vi "Voltage-Trans Converter.vi"(8 "Input":dbl, 9 "VoltageTransmissionArray":dbl[][](array[numeric]), 11 "Input":enum16{"Transmission", "Voltage"}(ring)) -> (1 "NearestTransmission":dbl, 3 "NearestVoltage":dbl)   [LabVIEW 2020]
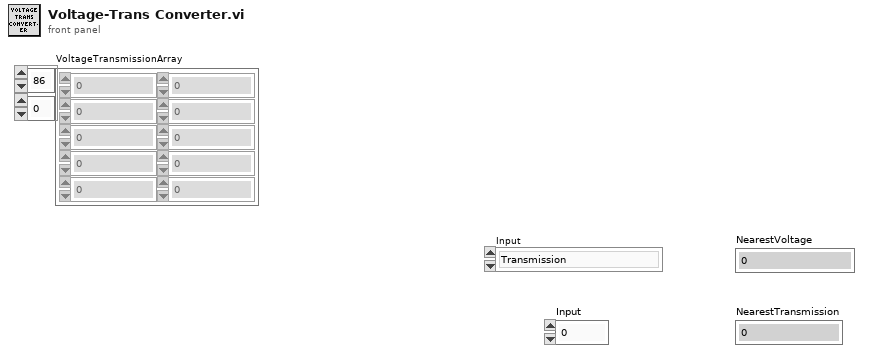
[diagram p1: front panel]
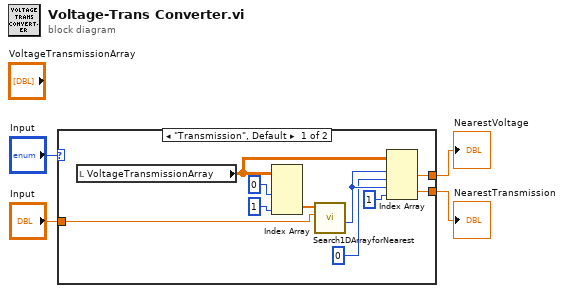
[diagram p0: block diagram]
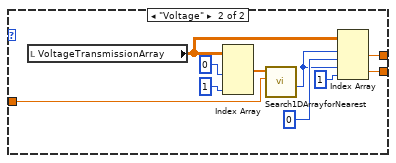
[diagram p2: hidden frame]
diagram:
  n1 = case shown="\"Transmission\", Default" "Input" {
    tunnel: "Input" -> [w8 w21]
    tunnel: [w7 w16] -> w1
    tunnel: [w6 w15] -> w2
    frame "Transmission", Default {
      n2 = local read "VoltageTransmissionArray"() -> (w14:dbl[][])
      n3 = Index Array(array=w14, index (col) #1=0 ("disabled index (col)"), index (col) #2=1 ("index (col)")) -> (element #2=w5:dbl[])  [unwired: 2 in, 1 out]
      n4 = call "Search1DArrayforNearest.vi"("desired element"=w8, "1D Array"=w5) -> ("closest index"=w13:i32)  [unwired: 8 in, 1 out]
      n5 = Index Array(array=w14, index (row) #1=w13, index (col) #1=0 ("disabled index (col)"), index (row) #2=w13, index (col) #2=1 ("index (col)")) -> (element #1=w7:dbl, element #2=w6:dbl)
    }
    frame "Voltage" {
      n6 = local read "VoltageTransmissionArray"() -> (w20:dbl[][])
      n7 = Index Array(array=w20, index (col) #1=0 ("disabled index (col)"), index (col) #2=1 ("index (col)")) -> (element #1=w22:dbl[])  [unwired: 2 in, 1 out]
      n8 = call "Search1DArrayforNearest.vi"("desired element"=w21, "1D Array"=w22) -> ("closest index"=w17:i32)  [unwired: 8 in, 1 out]
      n9 = Index Array(array=w20, index (row) #1=w17, index (col) #1=0 ("disabled index (col)"), index (row) #2=w17, index (col) #2=1 ("index (col)")) -> (element #1=w16:dbl, element #2=w15:dbl)
    }
  }
  "NearestVoltage" <- w1
  "NearestTransmission" <- w2
